vi "PSDATA_Variant To ArrayAWFM.vi"(9 "error in":errorcluster, 10 "Value":variant) -> (1 "error out":errorcluster, 2 "Value":string, 4 "ArrayAWFM":waveform(dbl)[](graph))   [LabVIEW 2016]
doc: "Developer：YDX"
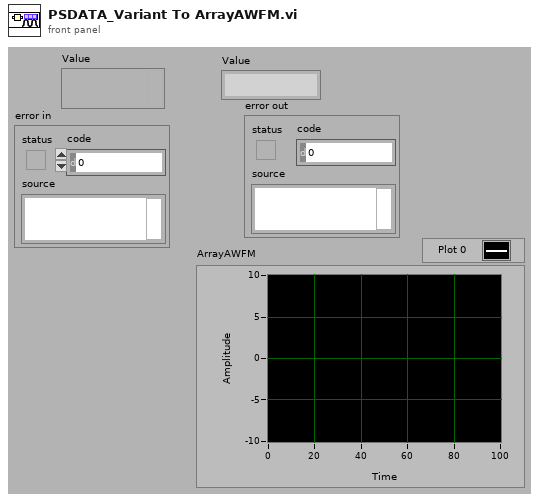
[diagram p1: front panel]
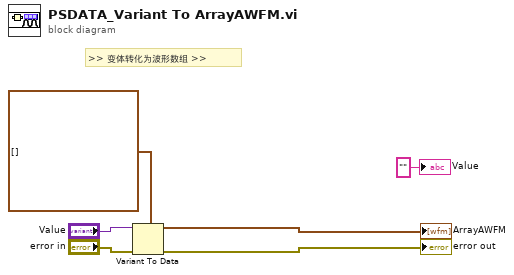
[diagram p0: block diagram]
diagram:
  # ">> 变体转化为波形数组 >>"
  n1 = Variant To Data(error in="error in", type=waveform(dbl)[] [], Variant="Value") -> (data=→"ArrayAWFM":waveform(dbl)[], error out=→"error out":errorcluster)
  "Value" <- "" ("Value")
